vi "Actor Core.vi"(8 "error in":errorcluster, 11 "UPNCalculatorGUI":refnum<class "UPNCalculatorGUI.lvclass">) -> (0 "error out":errorcluster, 3 "Actor out":refnum<class "Actor.lvclass">)   [LabVIEW 2012, in "UPNCalculatorGUI Actor.lvlib" / "UPNCalculatorGUI.lvclass"]
doc: "This is Actor Core.vi, the main message handling loop for Actors. An actor usually just sits in this loop and processes messages as they arrive. Any error returned by the message Do.vi call will stop the loop, with error code 43 as the canonical signal to stop with no error sent to caller. Descendants may override that in Handle Error.vi."
uses:
  UPNCalculatorGUI.lvclass
  <vilib>/ActorFramework/Actor/Actor.lvclass
  UPNCalculator Actor/UPNCalculator/UPNCalculator.lvclass
  <vilib>/ActorFramework/Actor/Actor.lvclass/Actor.ctl
  <vilib>/ActorFramework/Message Enqueuer/Message Enqueuer.lvclass/Message Enqueuer.ctl
  UPNCalculatorGUI.lvclass/UPNCalculatorGUI.ctl
  Calculator/Log Event Msg/Log Event Msg.lvclass/Log Event Msg.ctl
  UPNCalculator Actor/UPNCalculator Messages/Push Msg/Push Msg.lvclass/Push Msg.ctl
  UPNCalculator Actor/UPNCalculator Messages/Preview Stack Msg/Preview Stack Msg.lvclass/Preview Stack Msg.ctl
  <vilib>/ActorFramework/Message Enqueuer/Init from Existing Queue.vi
  <vilib>/ActorFramework/Message Enqueuer/Enqueue.vi
  <vilib>/ActorFramework/Message Priority Queue/Priority Enqueue.vi
  <vilib>/ActorFramework/Message Enqueuer/Message Enqueuer.lvclass
  Calculator/Log Event Msg/Log Event Msg.lvclass
  UPNCalculator Actor/UPNCalculator Messages/Push Msg/Push Msg.lvclass
  UPNCalculator Actor/UPNCalculator Messages/Preview Stack Msg/Preview Stack Msg.lvclass
  UPNCalculator Actor/UPNCalculator Messages/Pop Msg/Pop Msg.lvclass
  UPNCalculator Actor/UPNCalculator Messages/Flush Msg/Flush Msg.lvclass
  UPNCalculator Actor/UPNCalculator Messages/Add Msg/Add Msg.lvclass
  UPNCalculator Actor/UPNCalculator Messages/Substract Msg/Substract Msg.lvclass
panel:
  in  "Refresh":bool
  in  "Stack Preview":dbl[](array[numeric])
  in  "Clear":bool
  in  "Drop":bool
  in  "Enter":bool
  in  "Substract":bool
  in  "Add":bool
  in  "Input / Stack[0]":dbl
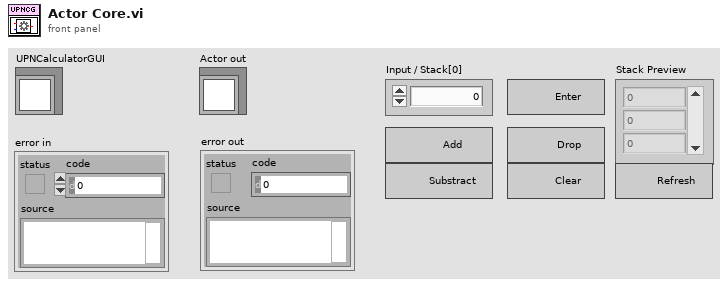
[diagram p1: front panel]
types:
  T1 = enum32{"Invalid", "Standard", "Closed", "Hidden", "Minimized", "Maximized"}
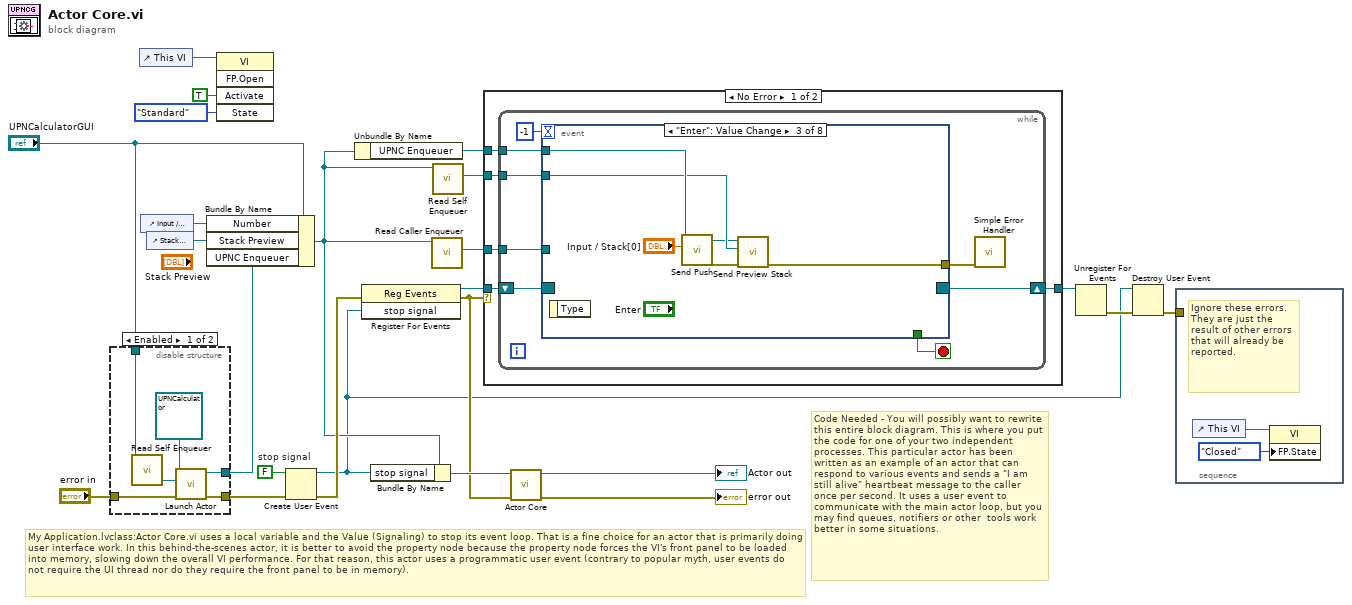
[diagram p0: block diagram]
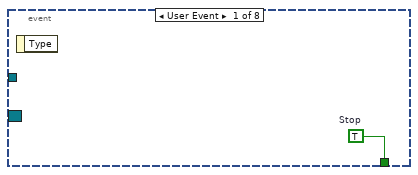
[diagram p3: hidden frame]
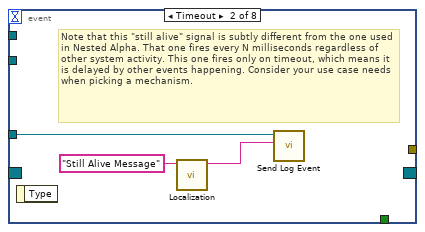
[diagram p4: hidden frame]
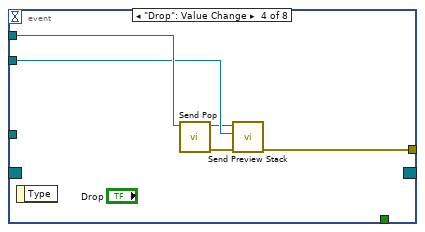
[diagram p5: hidden frame]
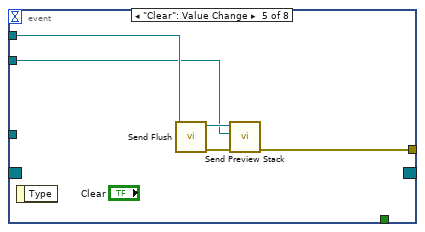
[diagram p6: hidden frame]
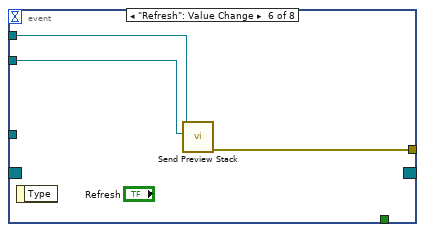
[diagram p7: hidden frame]
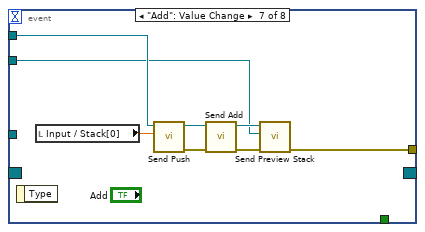
[diagram p8: hidden frame]
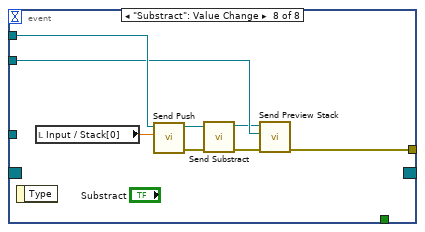
[diagram p9: hidden frame]
diagram:
  w21 = FALSE  # stop signal
  # "My Application.lvclass:Actor Core.vi uses a local variable and the Value (Signaling) to stop its event loop. That is a fine choice for an actor that is primarily doing user interface work. In this behind-the-scenes actor, it is better to avoid the property node because the property node forces the VI's front panel to be loaded into memory, slowing down the overall VI performance. For that reason, this actor uses a programmatic user event (contrary to popular myth, user events do not require the UI thread nor do they require the front panel to be in memory)."
  # "Code Needed - You will possibly want to rewrite this entire block diagram. This is where you put the code for one of your two independent processes. This particular actor has been written as an example of an actor that can respond to various events and sends a \"I am still alive\" heartbeat message to the caller once per second. It uses a user event to communicate with the main actor loop, but you may find queues, notifiers or other  tools work better in some situations."
  n1 = disable-structure shown="Enabled" {
    disable-tunnel: "UPNCalculatorGUI" -> [w30 _]
    disable-tunnel: "error in" -> [w28 w31]
    disable-tunnel: [w27 w31] -> w4
    disable-tunnel: [w26 _] -> w1
    frame Enabled {
      n2 = call <vilib>:"Read Self Enqueuer.vi"("Actor"=w30) -> ("Self Enqueuer"=w29:refnum<class "Message Enqueuer.lvclass">)  [unwired: 10 in]
      n3 = call <vilib>:"Launch Actor.vi"("error in (no error)"=w28, "Actor-to-Caller Enqueuer"=w29, "Actor"=refnum<class "UPNCalculator.lvclass"> refnum ("UPNCalculator Actor.lvlib:UPNCalculator.lvclass")) -> ("error out"=w27:errorcluster, "Caller-To-Actor Enqueuer"=w26:refnum<class "Message Enqueuer.lvclass">)  [unwired: 7 in]
    }
    frame Disabled {
    }
  }
  n4 = control-ref of="This VI"() -> (w9:refnum<vi>)
  n5 = control-ref of="Input / Stack[0]"() -> (w13:refnum<vi>)
  n6 = control-ref of="Stack Preview"() -> (w12:refnum<vi>)
  n7 = Bundle By Name(cluster="UPNCalculatorGUI", "Number"=w13, "Stack Preview"=w12, "UPNC Enqueuer"=w1) -> (w11:refnum<class "UPNCalculatorGUI.lvclass">)
  n8 = invoke class="VI" method="FP.Open"(reference=w9, "Activate"=TRUE ("Activate?"), "State"=T1."Standard") -> ()  [unwired: 2 in, 5 out]
  n9 = Create User Event(user event datatype=w21, error in=w4) -> (user event=w3:refnum<user-event>, error out=w20:errorcluster)
  n10 = Unbundle By Name(w11) -> ("UPNC Enqueuer"=w10:refnum<class "Message Enqueuer.lvclass">)
  n11 = register-events(error in=w20, w3) -> (reference out=w19:refnum<event-registration>, error out=w15:errorcluster)  [unwired: 1 in]
  n12 = Bundle By Name(cluster=w11, "stop signal"=w3) -> (w18:refnum<class "UPNCalculatorGUI.lvclass">)
  n13 = call <vilib>:"Read Caller Enqueuer.vi"("Actor"=w11) -> ("Caller Enqueuer"=w22:refnum<class "Message Enqueuer.lvclass">)  [unwired: 10 in]
  n14 = call <vilib>:"Read Self Enqueuer.vi"("Actor"=w11) -> ("Self Enqueuer"=w23:refnum<class "Message Enqueuer.lvclass">)  [unwired: 10 in]
  n15 = case shown="No Error" w15 {
    tunnel: w23 -> [w36 _]
    tunnel: w22 -> [w35 _]
    tunnel: w19 -> [w34 w84]
    tunnel: [w33 w84] -> w16
    tunnel: w10 -> [w32 _]
    frame No Error {
      n16 = while {
        tunnel: w36 -> [w43]
        tunnel: w35 -> [w42]
        shift-right: [w39] -> w33
        shift-left: w34 -> [w40]
        tunnel: w32 -> [w38]
        stop <- w44 stop-if-true
        n17 = event shown="[2] \"Enter\": Value Change" {
          selector: w40 -> [_ _ _ _ _ _ _ _]
          dyn-events: [_ _ _ _ _ _ _ _] -> w39
          timeout: -1 -> [_ _ _ _ _ _ _ _]
          tunnel: [w45 _ _ _ _ _ _ _] -> w44
          tunnel: w43 -> [_ _ w50 w57 w60 w65 w69 w81]
          tunnel: w42 -> [_ w48 _ _ _ _ _ _]
          tunnel: w38 -> [_ _ w51 w59 w64 w67 w75 w83]
          tunnel: [_ _ w52 w56 w61 w66 w68 w80] -> w37
          event User Event {
            w45 = TRUE  # Stop
            n18 = event-data() -> ()  [unwired: 1 in, 1 out]
          }
          event Timeout {
            # "Note that this \"still alive\" signal is subtly different from the one used in Nested Alpha. That one fires every N milliseconds regardless of other system activity. This one fires only on timeout, which means it is delayed by other events happening. Consider your use case needs when picking a mechanism."
            n19 = event-data() -> ()  [unwired: 1 in, 1 out]
            n20 = call "Localization.vi"("Unlocalized"="Still Alive Message") -> ("Localized"=w46:string)  [unwired: 10 in]
            n21 = call "Send Log Event.vi"("Event Text"=w46, "Message Enqueuer"=w48) -> ()  [unwired: 9 in, 1 out]
          }
          event "Enter": Value Change {
            n22 = event-data() -> ()  [unwired: 1 in, 1 out]
            n23 = call "Send Push.vi"("Element"="Input / Stack[0]", "Message Enqueuer"=w51) -> ("error out"=w53:errorcluster, "Message Enqueuer out"=w49:refnum<class "Message Enqueuer.lvclass">)  [unwired: 8 in]
            n24 = call "Send Preview Stack.vi"("error in (no error)"=w53, "Self Enqueuer"=w50, "Message Enqueuer"=w49) -> ("error out"=w52:errorcluster)  [unwired: 7 in, 1 out]
          }
          event "Drop": Value Change {
            n25 = event-data() -> ()  [unwired: 1 in, 1 out]
            n26 = call "Send Pop.vi"("Message Enqueuer"=w59) -> ("error out"=w58:errorcluster, "Message Enqueuer out"=w55:refnum<class "Message Enqueuer.lvclass">)  [unwired: 9 in]
            n27 = call "Send Preview Stack.vi"("error in (no error)"=w58, "Self Enqueuer"=w57, "Message Enqueuer"=w55) -> ("error out"=w56:errorcluster)  [unwired: 7 in, 1 out]
          }
          event "Clear": Value Change {
            n28 = event-data() -> ()  [unwired: 1 in, 1 out]
            n29 = call "Send Flush.vi"("Message Enqueuer"=w64) -> ("error out"=w62:errorcluster, "Message Enqueuer out"=w63:refnum<class "Message Enqueuer.lvclass">)  [unwired: 9 in]
            n30 = call "Send Preview Stack.vi"("error in (no error)"=w62, "Self Enqueuer"=w60, "Message Enqueuer"=w63) -> ("error out"=w61:errorcluster)  [unwired: 7 in, 1 out]
          }
          event "Refresh": Value Change {
            n31 = event-data() -> ()  [unwired: 1 in, 1 out]
            n32 = call "Send Preview Stack.vi"("Self Enqueuer"=w65, "Message Enqueuer"=w67) -> ("error out"=w66:errorcluster)  [unwired: 8 in, 1 out]
          }
          event "Add": Value Change {
            n33 = event-data() -> ()  [unwired: 1 in, 1 out]
            n34 = local read "Input / Stack[0]"() -> (w74:dbl)
            n35 = call "Send Push.vi"("Element"=w74, "Message Enqueuer"=w75) -> ("error out"=w72:errorcluster, "Message Enqueuer out"=w73:refnum<class "Message Enqueuer.lvclass">)  [unwired: 8 in]
            n36 = call "Send Add.vi"("error in (no error)"=w72, "Message Enqueuer"=w73) -> ("error out"=w70:errorcluster, "Message Enqueuer out"=w71:refnum<class "Message Enqueuer.lvclass">)  [unwired: 8 in]
            n37 = call "Send Preview Stack.vi"("error in (no error)"=w70, "Self Enqueuer"=w69, "Message Enqueuer"=w71) -> ("error out"=w68:errorcluster)  [unwired: 7 in, 1 out]
          }
          event "Substract": Value Change {
            n38 = event-data() -> ()  [unwired: 1 in, 1 out]
            n39 = local read "Input / Stack[0]"() -> (w82:dbl)
            n40 = call "Send Push.vi"("Element"=w82, "Message Enqueuer"=w83) -> ("error out"=w78:errorcluster, "Message Enqueuer out"=w79:refnum<class "Message Enqueuer.lvclass">)  [unwired: 8 in]
            n41 = call "Send Substract.vi"("error in (no error)"=w78, "Message Enqueuer"=w79) -> ("error out"=w77:errorcluster, "Message Enqueuer out"=w76:refnum<class "Message Enqueuer.lvclass">)  [unwired: 8 in]
            n42 = call "Send Preview Stack.vi"("error in (no error)"=w77, "Self Enqueuer"=w81, "Message Enqueuer"=w76) -> ("error out"=w80:errorcluster)  [unwired: 7 in, 1 out]
          }
        }
        n43 = call <vilib>:"Simple Error Handler.vi"("error in (no error)"=w37) -> ()  [unwired: 4 in, 5 out]
      }
    }
    frame Error {
    }
  }
  n44 = call-parent "Actor Core.vi"("error in"=w15, "Actor in"=w18) -> ("error out"=→"error out":errorcluster, "Actor out"=→"Actor out":refnum<class "Actor.lvclass">)  [unwired: 8 in]
  n45 = Unregister For Events(event registration refnum=w16) -> (error out=w17:errorcluster)  [unwired: 1 in]
  n46 = Destroy User Event(user event=w3, error in=w17) -> (error out=w14:errorcluster)
  n47 = stacked-sequence {
    tunnel: w14 -> [_]
    frame #0 {
      # "Ignore these errors.\nThey are just the result of other errors that will already be reported."
      n48 = control-ref of="This VI"() -> (w85:refnum<vi>)
      n49 = property class="VI"(reference=w85, "FP.State"=T1."Closed" ("Front Panel Window:State")) -> ()  [unwired: 1 in, 2 out]
    }
  }
